vi "Load BG Image from File.vi"(8 "error in (no error)":errorcluster, 10 "BG Image Path":path, 11 "HIJ Vision Camera App in":refnum<class "HIJ Vision Camera App.lvclass">) -> (0 "error out":errorcluster, 3 "HIJ Vision Camera App out":refnum<class "HIJ Vision Camera App.lvclass">)   [LabVIEW 2020, in "HIJ Vision Camera App.lvlib" / "HIJ Vision Camera App.lvclass"]
uses:
  HIJ Vision Camera App.lvclass
  HIJ Vision Camera App.lvclass/HIJ Vision Camera App.ctl
  Display Actors/HIJ IMAQdx Display/HIJ IMAQdx Display Messages/Write BG Image Ref Msg/Write BG Image Ref Msg.lvclass
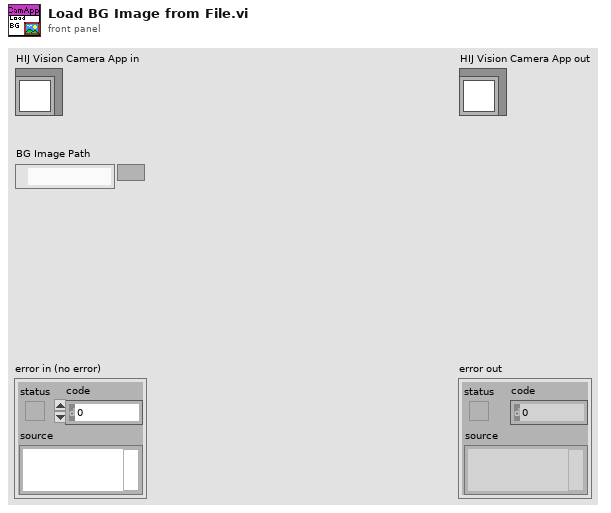
[diagram p1: front panel]
types:
  T1 = typedef "IMAQ Image.ctl" = refnum<image>
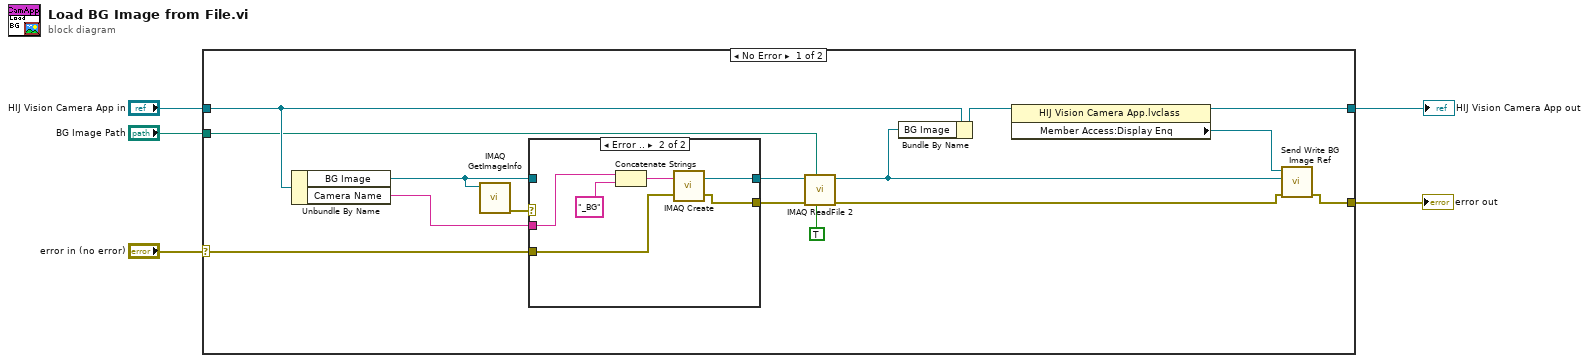
[diagram p0: block diagram]
diagram:
  n1 = case shown="No Error" "error in (no error)" {
    selector: "error in (no error)" -> [w14 w30]
    tunnel: [w7 w30] -> w4
    tunnel: [w10 w29] -> w2
    tunnel: "HIJ Vision Camera App in" -> [w20 w29]
    tunnel: "BG Image Path" -> [w12 _]
    frame No Error {
      n2 = Unbundle By Name(w20) -> ("BG Image"=w17:T1, "Camera Name"=w18:string)
      n3 = call "IMAQ GetImageInfo"("Image"=w17) -> ("error out"=w19:errorcluster)  [unwired: 3 in, 7 out]
      n4 = case shown="Error .." w19 {
        tunnel: w18 -> [_ w28]
        tunnel: w17 -> [w22 _]
        tunnel: [w22 w25] -> w16
        tunnel: [w21 w24] -> w15
        tunnel: w14 -> [w21 w23]
        frame No Error {
        }
        frame Error {
          n5 = Concatenate Strings(w28, "_BG" ("string")) -> (w27:string)
          n6 = call "IMAQ Create"("Image Name"=w27, "error in (no error)"=w23) -> ("New Image"=w25:T1, "error out"=w24:errorcluster)  [unwired: 3 in]
        }
      }
      n7 = call "IMAQ ReadFile 2"("Use File Path Image Type"=TRUE, "File Path"=w12, "error in (no error)"=w15, "Image"=w16) -> ("error out"=w8:errorcluster, "Image Out"=w6:T1)  [unwired: 3 in, 3 out]
      n8 = Bundle By Name(cluster=w20, "BG Image"=w6) -> (w11:refnum<class "HIJ Vision Camera App.lvclass">)
      n9 = property class="HIJ Vision Camera App.lvclass"(reference=w11) -> (reference out=w10:refnum<class "HIJ Vision Camera App.lvclass">, "Member Access:Display Enq"=w9:refnum<class "Message Enqueuer.lvclass">)  [unwired: 1 in, 1 out]
      n10 = call "Send Write BG Image Ref.vi"("error in (no error)"=w8, "Image"=w6, "Message Enqueuer"=w9) -> ("error out"=w7:errorcluster)  [unwired: 7 in, 1 out]
    }
    frame Error {
    }
  }
  "error out" <- w4
  "HIJ Vision Camera App out" <- w2
